vi "test Queue Metadata.vi"(8 "error in (no error)":errorcluster, 11 "TestCase in":refnum<class "Test_Queue.lvclass">) -> (0 "error out":errorcluster, 3 "TestCase out":refnum<class "Test_Queue.lvclass">)   [LabVIEW 2015, in "Test_Queue.lvclass"]
uses:
  Test_Queue.lvclass
  Core/Name Value Pair.ctl
  Global Parameters.vi
  Core/Session/Session.lvclass
  Core/NI_Azure_Core.lvlib
  Queue/NI_Azure_Queue.lvlib
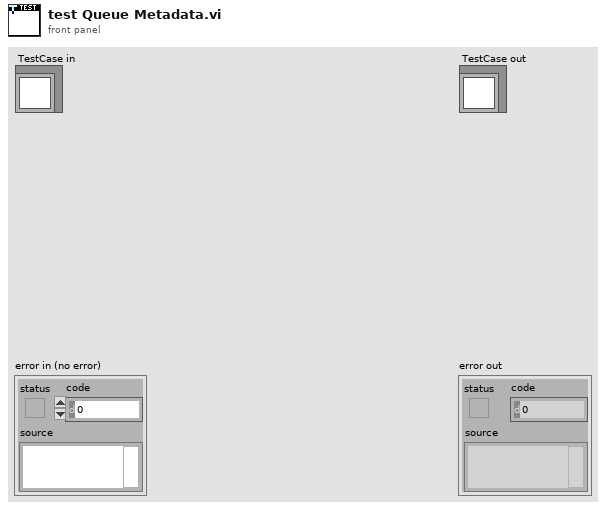
[diagram p1: front panel]
types:
  T1 = typedef "NI_Azure_Core.lvlib/Name Value Pair.ctl" = cluster{"name":string, "value":string}
  T2 = typedef "NI_Azure_Core.lvlib/Azure Credentials.ctl" = cluster{"Storage Account Name":string, "Access Key":string}
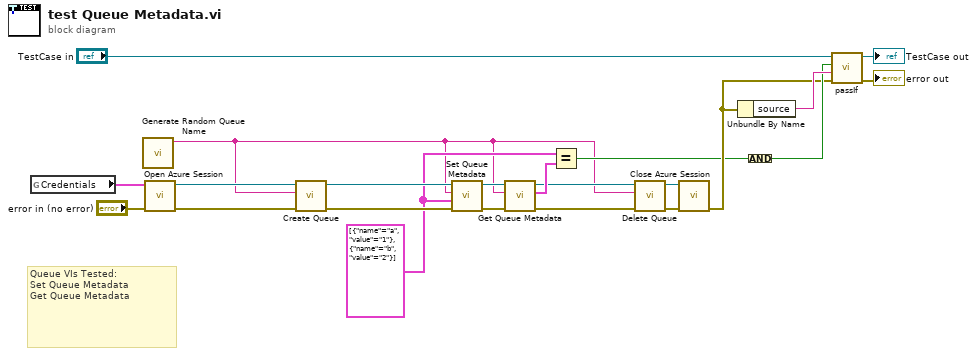
[diagram p0: block diagram]
diagram:
  w4 = T1[] [{"name"="a", "value"="1"}, {"name"="b", "value"="2"}] ("Metadata")
  # "Queue VIs Tested:\nSet Queue Metadata\nGet Queue Metadata"
  n1 = global read "Global Parameters.vi" "Credentials"() -> (w15:T2)
  n2 = call "Generate Random Queue Name.vi"() -> ("Random Queue Name"=w1:string)  [unwired: 11 in]
  n3 = call "Open Azure Session.vi"("error in (no error)"="error in (no error)", "Credentials"=w15) -> ("error out"=w16:errorcluster, "Azure Session"=w12:refnum<class "Session.lvclass">)  [unwired: 8 in]
  n4 = call "Create Queue.vi"("error in (no error)"=w16, "Queue"=w1, "Azure Session in"=w12) -> ("error out"=w18:errorcluster, "Azure Session out"=w8:refnum<class "Session.lvclass">)  [unwired: 7 in]
  n5 = call "Set Queue Metadata.vi"("error in (no error)"=w18, "Metadata"=w4, "Queue"=w1, "Azure Session in"=w8) -> ("error out"=w9:errorcluster, "Azure Session out"=w6:refnum<class "Session.lvclass">)  [unwired: 6 in]
  n6 = call "Get Queue Metadata.vi"("error in (no error)"=w9, "Queue"=w1, "Azure Session in"=w6) -> ("error out"=w7:errorcluster, "Metadata"=w5:T1[], "Azure Session out"=w2:refnum<class "Session.lvclass">)  [unwired: 6 in]
  n7 = Equal?(x=w4, y=w5) -> (x = y?=w3:bool)
  n8 = call "Delete Queue.vi"("error in (no error)"=w7, "Queue"=w1, "Azure Session in"=w2) -> ("error out"=w14:errorcluster, "Azure Session out"=w10:refnum<class "Session.lvclass">)  [unwired: 7 in]
  n9 = call "Close Azure Session.vi"("error in (no error)"=w14, "Azure Session"=w10) -> ("error out"=w11:errorcluster)  [unwired: 9 in]
  n10 = Unbundle By Name(w11) -> ("source"=w19:string)
  n11 = Compound Arithmetic op=AND(w3) -> (w13:bool)
  n12 = call-dynamic "passIf.vi"("error in (no error)"=w11, "message (\"\")"=w19, "pass"=w13, "TestCase in"="TestCase in") -> ("error out"=→"error out":errorcluster, "TestCase out"=→"TestCase out":refnum<class "Test_Queue.lvclass">)  [unwired: 6 in]
